vi "Close Caller FP if In LabVIEW folder.vi"(7 "VI Ref":refnum<vi>, 8 "error in (no error)":errorcluster) -> (0 "error out":errorcluster)   [LabVIEW 2017, in "csm_tool_menu.lvlib"]
doc: "lvAPT-User-Libraries 2022.4.27.213228\nYAO - lvAPT\nCopyright (c) 2022, lvAPT"
uses:
  csm_tool_menu.lvlib
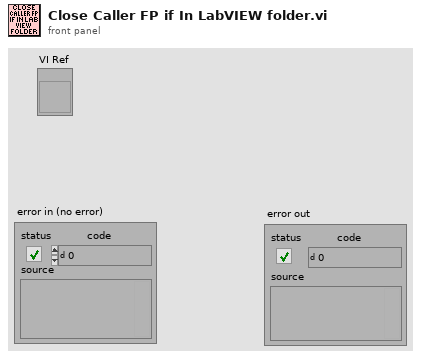
[diagram p1: front panel]
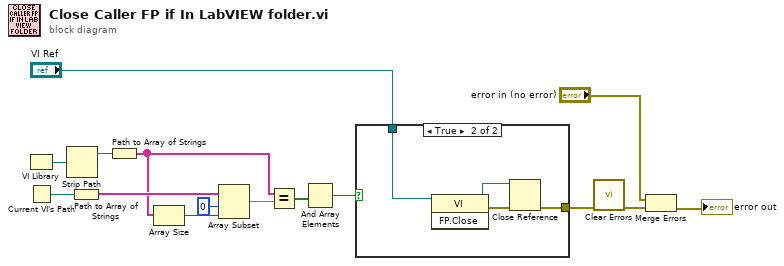
[diagram p0: block diagram]
diagram:
  n1 = VI Library() -> (path=w14:path)
  n2 = Current VI's Path() -> (path=w12:path)
  n3 = Strip Path(path=w14) -> (stripped path=w13:path)  [unwired: 1 out]
  n4 = Path to Array of Strings(0:w12) -> (2:w11:string[])  [unwired: 1 out]
  n5 = Path to Array of Strings(0:w13) -> (2:w7:string[])  [unwired: 1 out]
  n6 = Array Size(array=w7) -> (size(s)=w10:i32)
  n7 = Array Subset(array=w11, index=0, length=w10) -> (w8:string[])
  n8 = Equal?(x=w7, y=w8) -> (x = y?=w6:bool[])
  n9 = And Array Elements(Boolean array=w6) -> (logical AND=w5:bool)
  n10 = case shown="True" w5 {
    tunnel: [_ w18] -> w15
    tunnel: "VI Ref" -> [_ w16]
    frame False {
    }
    frame True {
      n11 = invoke class="VI" method="FP.Close"(reference=w16) -> (reference out=w17:refnum<vi>, error out=w19:errorcluster)  [unwired: 2 in, 1 out]
      n12 = Close Reference(reference=w17, error in (no error)=w19) -> (error out=w18:errorcluster)
    }
  }
  n13 = call <vilib>:"Clear Errors.vi"("error in (no error)"=w15) -> ("error out"=w2:errorcluster)  [unwired: 5 in, 1 out]
  n14 = Merge Errors("error in (no error)", w2) -> (→"error out":errorcluster)
